vi "Global 1.vi"() -> ()   [LabVIEW 2009]
panel:
  in  "printer":bool=TRUE
  in  "test path":T1
  in  "acceptance Limits":T2={"VHEATFUSENOLOADMIN"="4.40", "VHEATFUSELOADMAX"="2.00", "VOVERRIDEDIODEMIN"="3.25", "TDIFFMAX"="5", "MEASFREQMAX"="64.00288", "MEASFREQMIN"="63.99712", "VOVER"="3.60", "VMIDDLE"="3.40", "VUNDER"="3.20", "VNORESET"="2.85", "VRESET"="2.75", "WAITPING"="2", "LRFID"="2.0", "RFIDUID"="TAG_0459E071ED0280", "EXTEESIZE"="02", "LCUTYPE"="25", "LCUSUBTYPE"="00", "TEVN"="61", "BOOTVER"="BL 6331 V1.01       ", "APPVER"="104  LCU 6330/6331     ", "ISLEEPMAX"="15", "TSLEEP"="10", "APPWAIT"="2", "DBWAIT"="3"}
  in  "Print":refnum<visa-resource-name>="LPT1"
  in  "Product serial number":T3={"serial number"="", "Part number"="4821683", "Revision letter "="01", "Revision counter"="000", "Manufature"="005", "Year Week"=""}
  out "Write  S":T4
  in  "EXCLE path":string="F:\\Testdata\\LCU6331\\LCU 6331 EXCEL\\"
  in  "Txt path":string="F:\\Testdata\\LCU6331\\LCU6331 txt\\"
  out "Record":T4={"People"="", "product  number"="", "Test time"="", "VHeatFuse_noload"="", "VHeatFuse_load"="", "VoverrideDiode"="", "Test firmware upload via X1"="", "TemperAddress"="", "Troom"="", "TLCU"="", "Adjustment factor"="", "MeasuredFreq"="", "I2C communication"="", "Light-emitting diode on Z2"="", "Battery warning/inhibit"="", "Reset by IC10"="", "External EEPROM"="", "RFID card detection and reading RFID"="\n\n", "Production parameters in internal EEPROM"="", "Current consumption in sleep mode"="", "Application and database upload"="", "Test result"="", "Table head[22]"="", "Table head[23]"=""}
  in  "Freq 53131A":u32=3
  in  "UutPort":refnum<visa-resource-name>="COM1"
  in  "USB4065":refnum<k15>="Dev2"
  in  "Power E3631A":i32=5
  # "com3"
  # "com4"
  # "com1"
  # "Dev2"
  # "3"
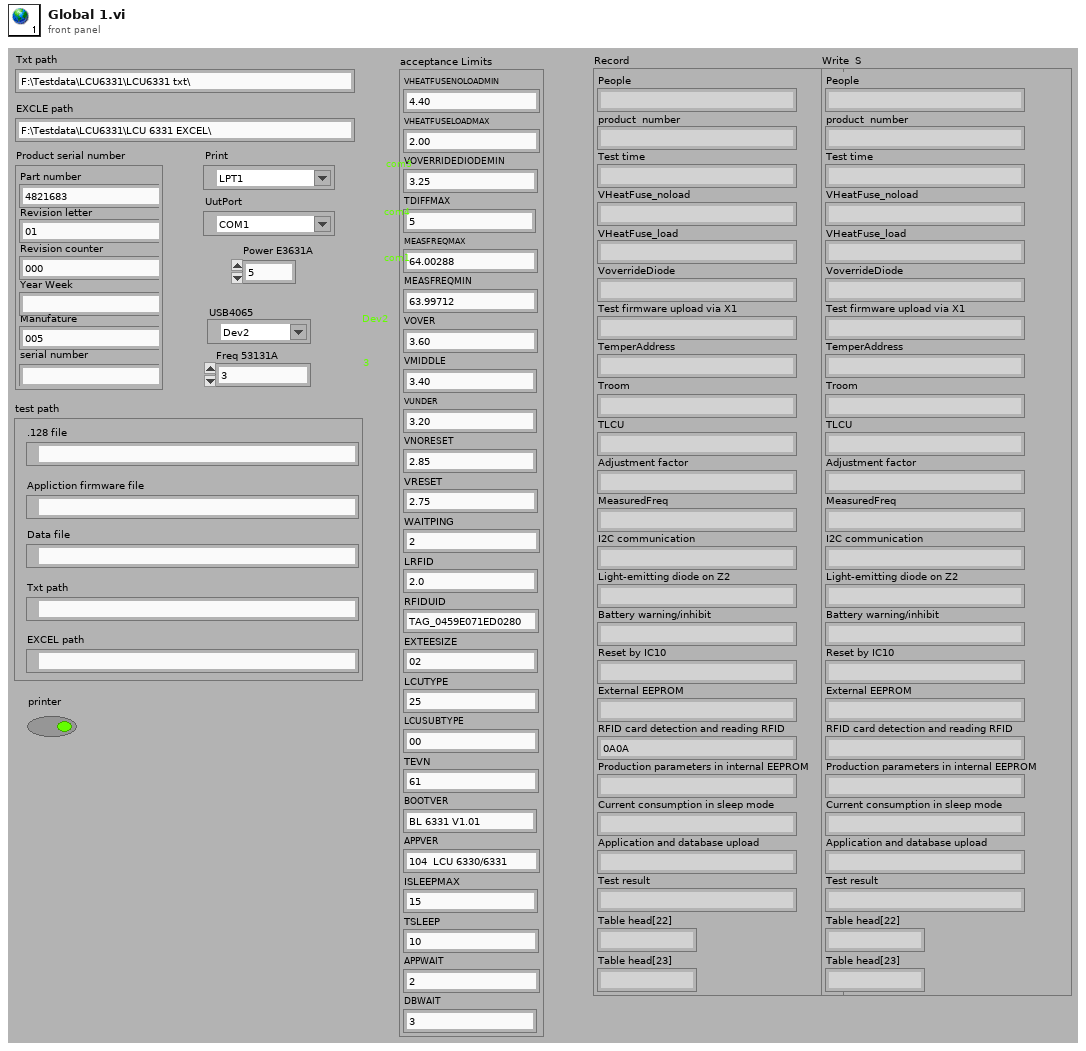
[diagram p1: front panel]
types:
  T1 = cluster{".128 file":path, "Appliction firmware file":path, "Data file":path, "Txt path":path, "EXCEL path":path}
  T2 = cluster{"VHEATFUSENOLOADMIN":string, "VHEATFUSELOADMAX":string, "VOVERRIDEDIODEMIN":string, "TDIFFMAX":string, "MEASFREQMAX":string, "MEASFREQMIN":string, "VOVER":string, "VMIDDLE":string, "VUNDER":string, "VNORESET":string, "VRESET":string, "WAITPING":string, "LRFID":string, "RFIDUID":string, "EXTEESIZE":string, "LCUTYPE":string, "LCUSUBTYPE":string, "TEVN":string, "BOOTVER":string, "APPVER":string, "ISLEEPMAX":string, "TSLEEP":string, "APPWAIT":string, "DBWAIT":string}
  T3 = cluster{"serial number":string, "Part number":string, "Revision letter ":string, "Revision counter":string, "Manufature":string, "Year Week":string}
  T4 = cluster{"People":string, "product  number":string, "Test time":string, "VHeatFuse_noload":string, "VHeatFuse_load":string, "VoverrideDiode":string, "Test firmware upload via X1":string, "TemperAddress":string, "Troom":string, "TLCU":string, "Adjustment factor":string, "MeasuredFreq":string, "I2C communication":string, "Light-emitting diode on Z2":string, "Battery warning/inhibit":string, "Reset by IC10":string, "External EEPROM":string, "RFID card detection and reading RFID":string, "Production parameters in internal EEPROM":string, "Current consumption in sleep mode":string, "Application and database upload":string, "Test result":string, "Table head[22]":string, "Table head[23]":string}
diagram:
